vi "Lin_Rohner_Project.vi"() -> ()   [LabVIEW 2019]
uses:
  <vilib>/Platform/TimedLoop/XDataNode/timing_clust.ctl
  <vilib>/Platform/TimedLoop/XDataNode/nitl_modes.ctl
  <vilib>/Platform/TimedLoop/XDataNode/wakeup.ctl
  <vilib>/Analysis/3filter.llb/Filter Passband Type.ctl
  <vilib>/DAQmx/write.llb/DAQmx Write (Analog DBL 1Chan 1Samp).vi
  <vilib>/DAQmx/read.llb/DAQmx Read (Analog 1D DBL NChan 1Samp).vi
  <vilib>/DAQmx/create/channels.llb/DAQmx Create Channel (AO-Voltage-Basic).vi
  <vilib>/DAQmx/miscellaneous.llb/DAQmx Fill In Error Info.vi
  <vilib>/DAQmx/create/channels.llb/DAQmx Create Channel (AI-Voltage-Basic).vi
  <vilib>/platform/TimedLoop/XDataNode/XDataNode.xnode
  <vilib>/Platform/TimedLoop/XDataNode/XDNodeRunTimeDep.lvlib
  <vilib>/ptbypt/NI_PtbyPt.lvlib
  <vilib>/Analysis/NI_AALBase.lvlib
panel:
  in  "Force Feedback":bool
  in  "Choose a Controller(Turn them ON first!!!)":bool
  out "Force Feedback Control Voltage":dbl
  out "Force Feedback Control Voltage":dbl(graph)
  in  "low cutoff freq: force sensor":dbl=0.125 format="%0.3f"
  out "Filtered Paddle Angular acce(tachometer) [rad/s^2]":dbl(graph)
  out "Filtered Paddle Angular acce(tachometer) [rad/s^2]":dbl
  in  "low cutoff freq: paddle angular acce":dbl=0.125 format="%0.3f"
  out "Filtered Torque [Nm]":dbl
  out "Filtered Torque [Nm]":dbl(graph)
  out "Filtered Paddle Angular Velocity(tachometer) [rad/s]":dbl
  out "Filtered Paddle Angular Velocity(tachometer) [rad/s] 2":dbl(graph)
  in  "low cutoff freq: paddle angular velocity(tachometer)":dbl=0.125 format="%0.3f"
  out "Angular Position [deg]":dbl
  out "Angular Position [deg]":dbl(knob) scale=-32.5..32.5
  in  "B":dbl
  in  "K":dbl
  in  "Virtual Wall":bool
  in  "Position Filter":bool
  out "Compensation Voltage":dbl
  out "Compensation Voltage":dbl(graph)
  out "Gravity Compesation":dbl
  out "Friction Compensation":dbl
  in  "Friction Compensation":bool
  in  "Gravaty Compensation":bool
  out "Friction Compensation":dbl(graph)
  out "Gravity Compesation":dbl(graph)
  in  "low cutoff freq: Position":dbl=0.125 format="%0.3f"
  in  "stop":bool
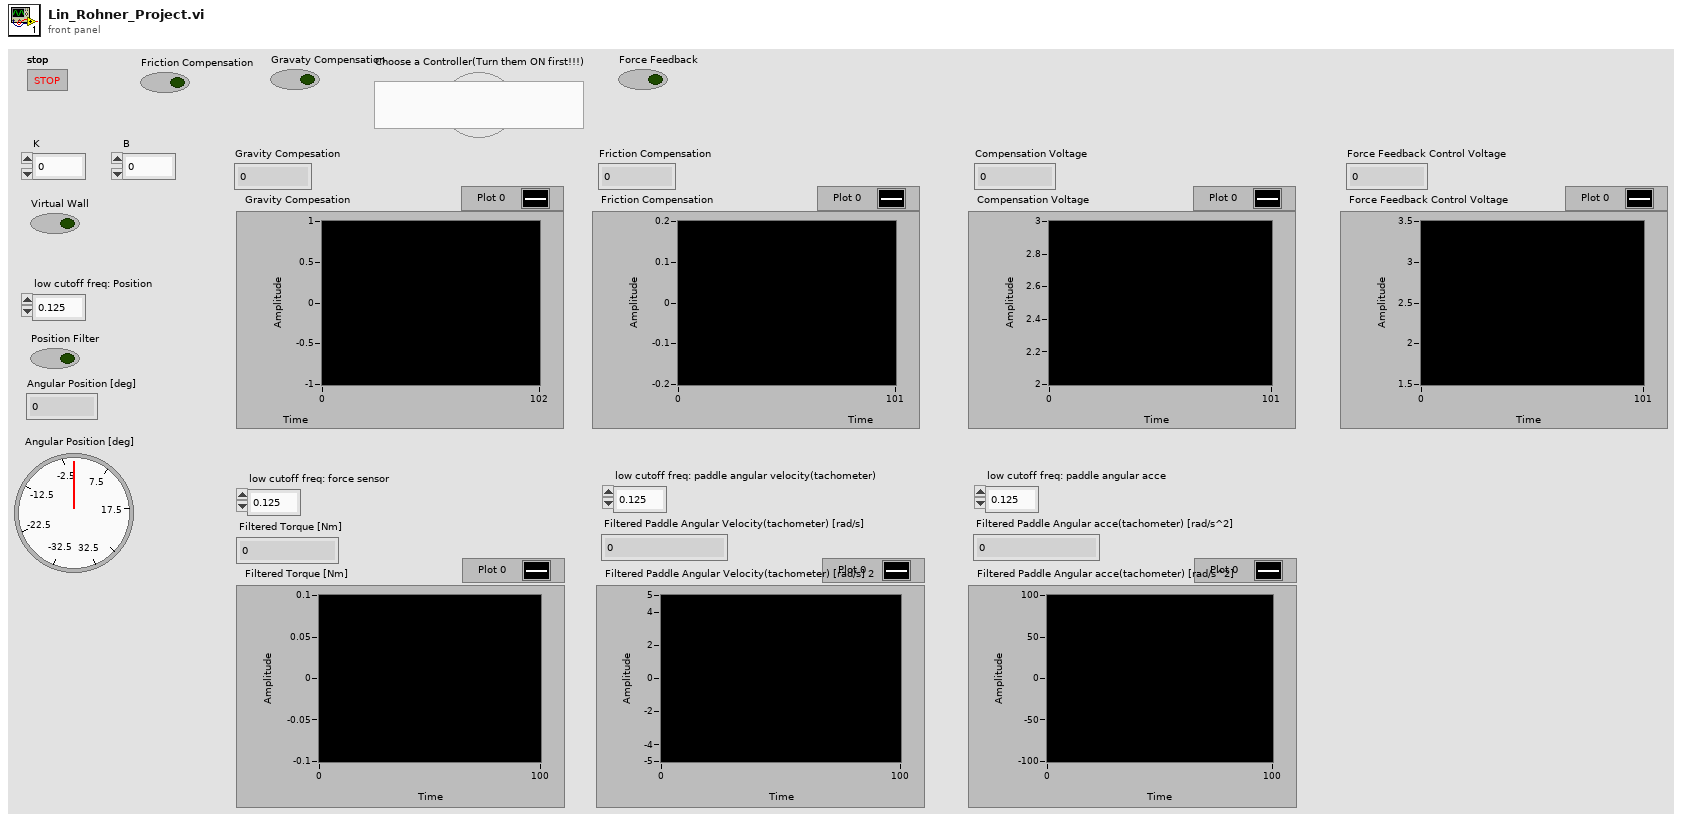
[diagram p1: front panel]
types:
  T1 = typedef "NI_AALBase.lvlib/Filter Passband Type.ctl" = enum32{"Lowpass", "Highpass", "Bandpass", "Bandstop"}
  T2 = typedef "XDNodeRunTimeDep.lvlib/timing_clust.ctl" = cluster{"Expected End [f-1]":u64, "Actual End [f-1]":u64, "Finished Late? [f-1]":bool, "Expected End [i-1]":u64, "Actual End [i-1]":u64, "Finished Late? [i-1]":bool, "Expected Start [i]":u64, "Actual Start [i]":u64, "Expected Start [f]":u64, "Actual Start [f]":u64, "Source Name":string, "Structure Name":string, "Period":i64, "Deadline":i64, "Offset":i64, "Start":i64, "Priority":i32, "Timeout":i32, "Mode":T3, "Wakeup Reason":T4, "Error":errorcluster, "Source Type":string, "Secondary Source Type":string, "Global End Time":u64, "Global Start Time":u64, "Frame Duration":u64, "Iteration Duration":u64, "Assigned CPU":i32, "I/O Scan Engine Mode":u32}
  T3 = typedef "XDNodeRunTimeDep.lvlib/nitl_modes.ctl" = enum32{"No Change", "Process missed periods, maintain original phase", "Discard missed periods, maintain original phase", "Process missed periods, ignore original phase", "Discard missed periods, ignore original phase"}
  T4 = typedef "XDNodeRunTimeDep.lvlib/wakeup.ctl" = enum32{"Normal", "Aborted", "Asynchronous wakeup", "Timing source error", "Timed loop error", "Timeout"}
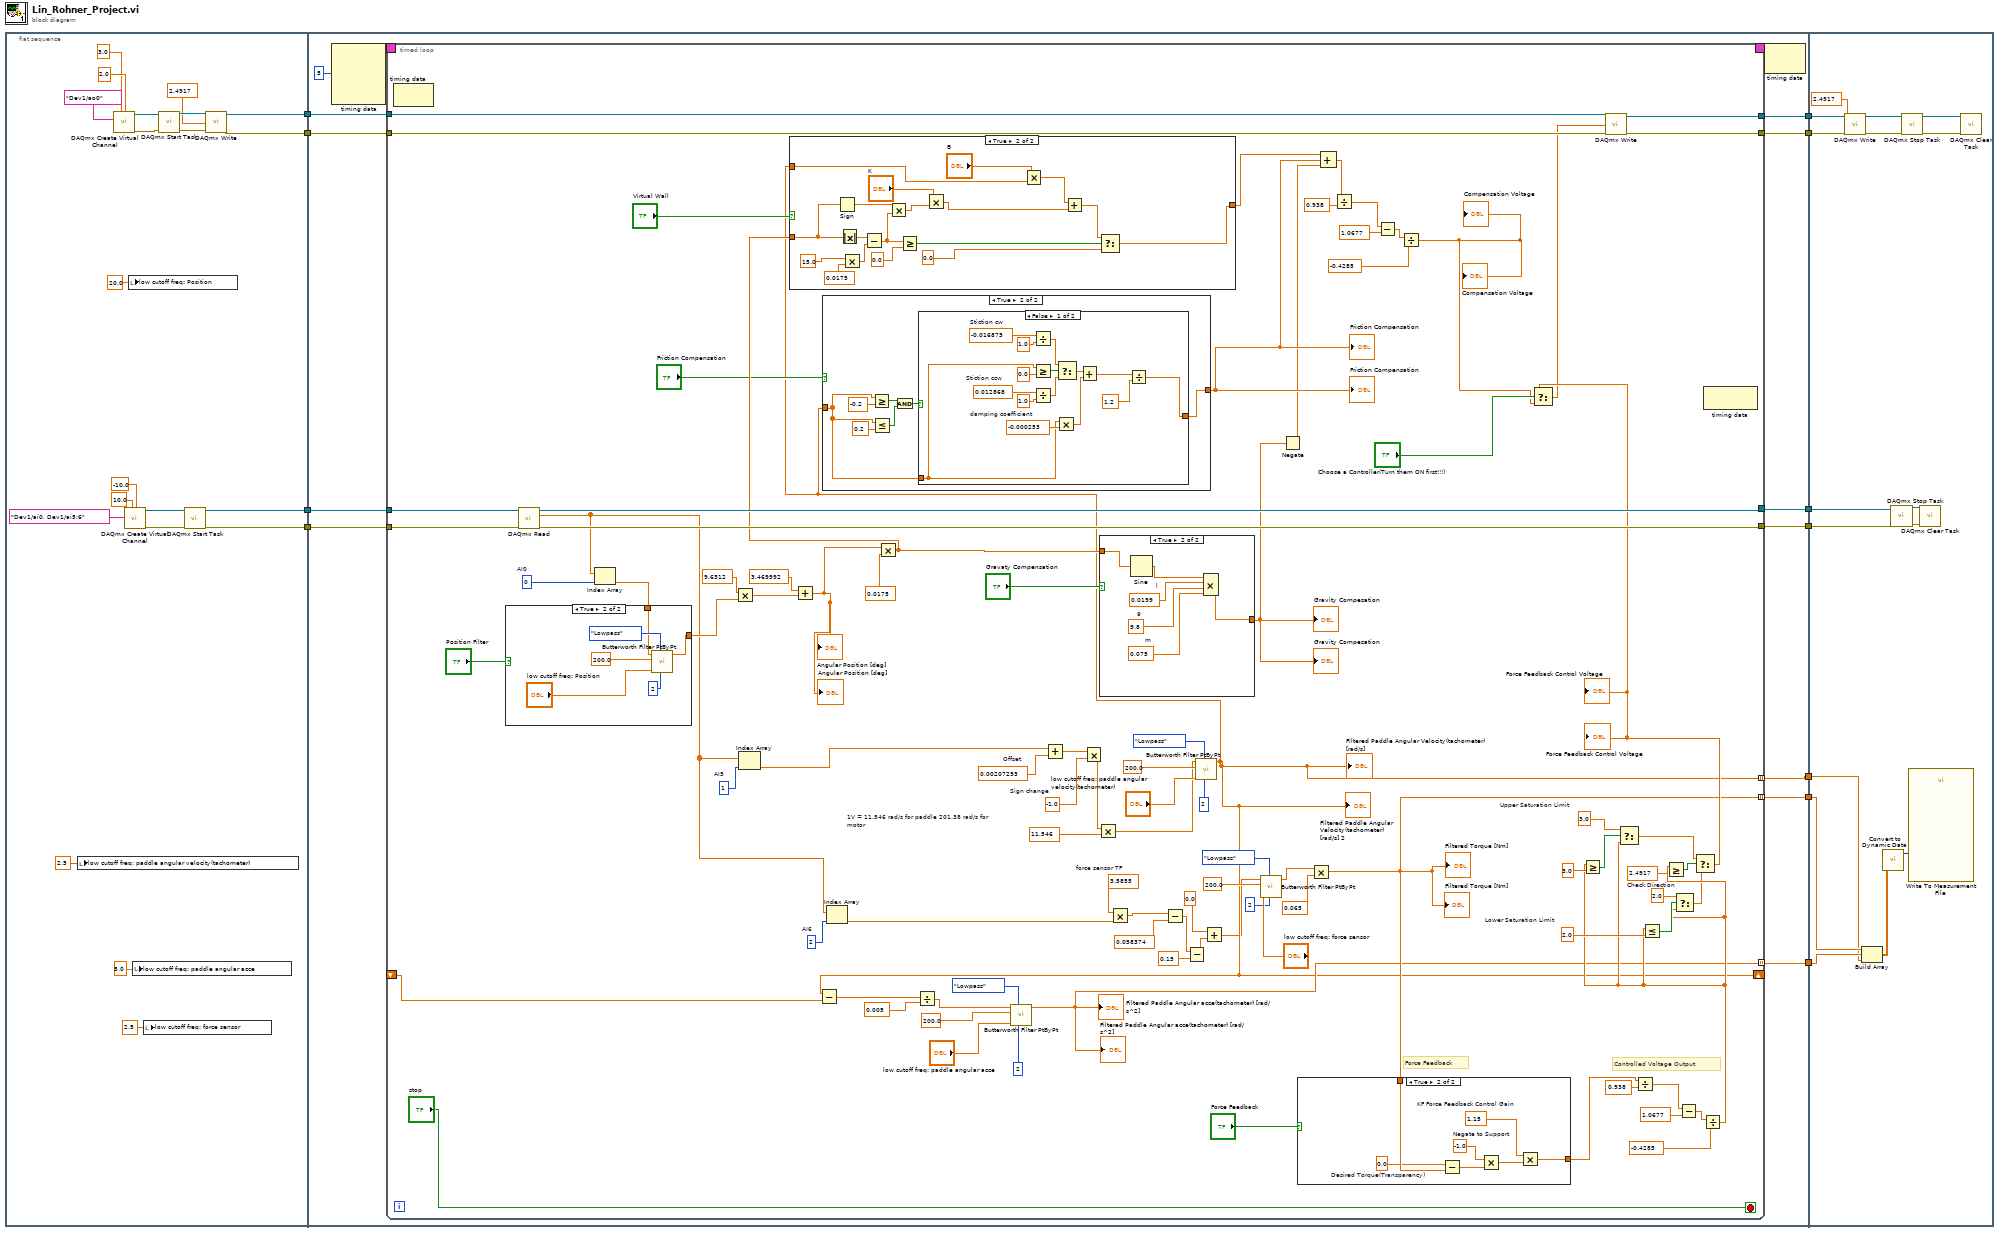
[diagram p0: block diagram]
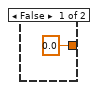
[diagram p2: hidden frame]
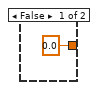
[diagram p3: hidden frame]
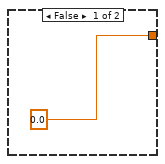
[diagram p5: hidden frame]
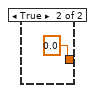
[diagram p6: hidden frame]
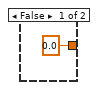
[diagram p7: hidden frame]
diagram:
  n1 = flat-sequence {
    tunnel: [w30] -> w11
    tunnel: [w29] -> w10
    tunnel: [w18] -> w9
    tunnel: [w17] -> w8
    tunnel: w11 -> [w43]
    tunnel: w10 -> [w42]
    tunnel: w9 -> [w41]
    tunnel: w8 -> [w40]
    tunnel: [w39] -> w7
    tunnel: [w38] -> w6
    tunnel: [w37] -> w5
    tunnel: [w36] -> w4
    tunnel: [w35] -> w3
    tunnel: [w34] -> w2
    tunnel: [w33] -> w1
    tunnel: w7 -> [w220]
    tunnel: w6 -> [w219]
    tunnel: w5 -> [w218]
    tunnel: w4 -> [w217]
    tunnel: w3 -> [w216]
    tunnel: w2 -> [w215]
    tunnel: w1 -> [w214]
    frame #0 {
      n2 = local write "low cutoff freq: paddle angular velocity(tachometer)"(2.5 ("low cutoff freq: paddle angular velocity(tachometer)")) -> ()
      n3 = call-poly <vilib>:"DAQmx Create Virtual Channel.vi"("maximum value"=3.0, "minimum value"=2.0, "physical channels"=tag "Dev1/ao0") -> ("task out"=w32:refnum<k21>, "error out"=w28:errorcluster)  [unwired: 11 in]
      n4 = call-poly <vilib>:"DAQmx Create Virtual Channel.vi"("maximum value"=10.0, "minimum value"=-10.0, "physical channels"=tag "Dev1/ai0, Dev1/ai5:6") -> ("task out"=w19:refnum<k21>, "error out"=w20:errorcluster)  [unwired: 11 in]
      n5 = local write "low cutoff freq: Position"(20.0 ("low cutoff freq: Position")) -> ()
      n6 = local write "low cutoff freq: paddle angular acce"(5.0 ("low cutoff freq: paddle angular acce")) -> ()
      n7 = local write "low cutoff freq: force sensor"(2.5 ("low cutoff freq: force sensor")) -> ()
      n8 = call <vilib>:"DAQmx Start Task.vi"("task/channels in"=w32, "error in"=w28) -> ("task out"=w31:refnum<k21>, "error out"=w27:errorcluster)  [unwired: 12 in]
      n9 = call <vilib>:"DAQmx Start Task.vi"("task/channels in"=w19, "error in"=w20) -> ("task out"=w18:refnum<k21>, "error out"=w17:errorcluster)  [unwired: 12 in]
      n10 = call-poly <vilib>:"DAQmx Write.vi"("task/channels in"=w31, "data"=2.4917, "error in"=w27) -> ("task out"=w30:refnum<k21>, "error out"=w29:errorcluster)  [unwired: 10 in, 1 out]
    }
    frame #1 {
      n11 = node-c288(i64 5 ("Period")) -> (w46:T2)  [unwired: 3 in]
      n12 = timed-loop {
        timing: w46 -> [_]
        timing-out: [_] -> w45
        tunnel: w43 -> [w136]
        tunnel: w42 -> [w135]
        tunnel: w41 -> [w134]
        tunnel: w40 -> [w133]
        tunnel: [w130] -> w39
        tunnel: [w129] -> w38
        tunnel: [w132] -> w37
        tunnel: [w131] -> w36
        shift-right: [w50] -> _
        shift-left: _ -> [w88]
        tunnel: [w52] -> w35 mode=indexing
        tunnel: [w51] -> w34 mode=indexing
        tunnel: [w50] -> w33 mode=indexing
        stop <- "stop" stop-if-true
        w61 = 2.4917  # Check Direction
        w65 = 2.0  # Lower Saturation Limit
        w68 = 3.0  # Upper Saturation Limit
        w94 = 3.5855  # force sensor TF
        w96 = 2  # AI6
        w103 = 11.546  # 1V = 11.546 rad/s for paddle 201.38 rad/s for motor
        w105 = -1.0  # Sign change
        w107 = 0.00207293  # Offset
        w109 = 1  # AI5
        w111 = 0  # AI0
        # "Controlled Voltage Output"
        # "Force Feedback"
        n13 = node-c288() -> ()  [unwired: 1 in, 1 out]
        n14 = call-poly <vilib>:"DAQmx Read.vi"("task/channels in"=w134, "error in"=w133) -> ("task out"=w132:refnum<k21>, "data"=w91:dbl[], "error out"=w131:errorcluster)  [unwired: 11 in]
        n15 = Index Array(array=w91, index=w111) -> (element=w110:dbl)
        n16 = case shown="True" "Position Filter" {
          tunnel: [w168 w171] -> w137
          tunnel: w110 -> [w168 w169]
          frame False {
          }
          frame True {
            n17 = call <vilib>:"Butterworth Filter PtByPt.vi"("order"=2, "filter type"=Filter_Passband_Type."Lowpass", "low cutoff freq: fl"="low cutoff freq: Position", "sampling freq: fs"=200.0, "x"=w169) -> ("Filtered x"=w171:dbl)  [unwired: 4 in, 1 out]
          }
        }
        n18 = Multiply(x=9.6312, y=w137) -> (x*y=w139:dbl)
        n19 = Index Array(array=w91, index=w109) -> (element=w108:dbl)
        n20 = Add(x=3.469992, y=w139) -> (x+y=w112:dbl)
        "Angular Position [deg]" <- w112
        "Angular Position [deg]" <- w112
        n21 = Index Array(array=w91, index=w96) -> (element=w95:dbl)
        n22 = Multiply(x=w112, y=0.0175) -> (x*y=w113:dbl)
        n23 = Add(x=w108, y=w107) -> (x+y=w106:dbl)
        n24 = Multiply(x=w106, y=w105) -> (x*y=w104:dbl)
        n25 = Multiply(x=w104, y=w103) -> (x*y=w98:dbl)
        n26 = case shown="True" "Gravaty Compensation" {
          tunnel: [0.0 w201] -> w120
          tunnel: w113 -> [_ w200]
          frame False {
          }
          frame True {
            w202 = 0.075  # m
            w203 = 9.8  # g
            w204 = 0.0199  # l
            n27 = Sine(x=w200) -> (sin(x)=w205:dbl)
            n28 = Compound Arithmetic op=MULTIPLY(w205, w204, w203, w202) -> (w201:dbl)
          }
        }
        "Gravity Compesation" <- w120
        "Gravity Compesation" <- w120
        n29 = Multiply(x=w94, y=w95) -> (x*y=w93:dbl)
        n30 = Subtract(x=w93, y=0.058374) -> (x-y=w89:dbl)
        n31 = Subtract(x=w89, y=0.15) -> (x-y=w49:dbl)
        n32 = call <vilib>:"Butterworth Filter PtByPt.vi"("order"=2, "filter type"=Filter_Passband_Type."Lowpass", "low cutoff freq: fl"="low cutoff freq: paddle angular velocity(tachometer)", "sampling freq: fs"=200.0, "x"=w98) -> ("Filtered x"=w50:dbl)  [unwired: 4 in, 1 out]
        "Filtered Paddle Angular Velocity(tachometer) [rad/s] 2" <- w50
        "Filtered Paddle Angular Velocity(tachometer) [rad/s]" <- w50
        n33 = case shown="True" "Virtual Wall" {
          tunnel: w113 -> [_ w163]
          tunnel: w50 -> [_ w159]
          tunnel: [0.0 w155] -> w115
          frame False {
          }
          frame True {
            n34 = Sign(1:w163) -> (0:w162:dbl)
            n35 = Absolute Value(x=w163) -> (abs(x)=w166:dbl)
            n36 = Multiply(x=15.0 ("y"), y=0.0175) -> (x*y=w150:dbl)
            n37 = Subtract(x=w166, y=w150) -> (x-y=w161:dbl)
            n38 = Multiply(x=w162, y=w161) -> (x*y=w160:dbl)
            n39 = Greater Or Equal?(x=w161, y=0.0) -> (x >= y?=w164:bool)
            n40 = Multiply(x="K", y=w160) -> (x*y=w157:dbl)
            n41 = Multiply(x="B", y=w159) -> (x*y=w158:dbl)
            n42 = Add(x=w158, y=w157) -> (x+y=w156:dbl)
            n43 = Select(t=w156, s=w164, f=0.0) -> (s? t:f=w155:dbl)
          }
        }
        n44 = Subtract(x=w50, y=w88) -> (x-y=w87:dbl)
        n45 = case shown="True" "Friction Compensation" {
          tunnel: [0.0 ("f") w177] -> w117
          tunnel: w50 -> [_ w176]
          frame False {
          }
          frame True {
            n46 = Greater Or Equal?(x=w176, y=-0.2) -> (x >= y?=w180:bool)
            n47 = Less Or Equal?(x=w176, y=0.2) -> (x <= y?=w179:bool)
            n48 = And(x=w180, y=w179) -> (x .and. y?=w178:bool)
            n49 = case shown="False" w178 {
              tunnel: [w184 0.0 ("y")] -> w177
              tunnel: w176 -> [w193 _]
              frame False {
                w195 = -0.000253  # damping coefficient
                w191 = 0.012868  # Stiction ccw
                w188 = -0.016875  # Stiction cw
                n50 = Divide(x=w188, y=1.0) -> (x/y=w187:dbl)
                n51 = Greater Or Equal?(x=w193, y=0.0) -> (x >= y?=w196:bool)
                n52 = Divide(x=w191, y=1.0) -> (x/y=w190:dbl)
                n53 = Multiply(x=w193, y=w195) -> (x*y=w194:dbl)
                n54 = Select(t=w187, s=w196, f=w190) -> (s? t:f=w192:dbl)
                n55 = Add(x=w192, y=w194) -> (x+y=w185:dbl)
                n56 = Divide(x=w185, y=1.2) -> (x/y=w184:dbl)
              }
              frame True {
              }
            }
          }
        }
        "Friction Compensation" <- w117
        "Friction Compensation" <- w117
        n57 = Divide(x=w87, y=0.005) -> (x/y=w85:dbl)
        n58 = call <vilib>:"Butterworth Filter PtByPt.vi"("order"=2, "filter type"=Filter_Passband_Type."Lowpass", "low cutoff freq: fl"="low cutoff freq: paddle angular acce", "sampling freq: fs"=200.0, "x"=w85) -> ("Filtered x"=w51:dbl)  [unwired: 4 in, 1 out]
        "Filtered Paddle Angular acce(tachometer) [rad/s^2]" <- w51
        "Filtered Paddle Angular acce(tachometer) [rad/s^2]" <- w51
        n59 = Add(x=0.0, y=w49) -> (x+y=w47:dbl)
        n60 = call <vilib>:"Butterworth Filter PtByPt.vi"("order"=2, "filter type"=Filter_Passband_Type."Lowpass", "low cutoff freq: fl"="low cutoff freq: force sensor", "sampling freq: fs"=200.0, "x"=w47) -> ("Filtered x"=w76:dbl)  [unwired: 4 in, 1 out]
        n61 = Negate(x=w120) -> (-x=w116:dbl)
        n62 = Multiply(x=w76, y=0.065) -> (x*y=w52:dbl)
        "Filtered Torque [Nm]" <- w52
        "Filtered Torque [Nm]" <- w52
        n63 = case shown="True" "Force Feedback" {
          tunnel: w52 -> [_ w148]
          tunnel: [0.0 w142] -> w69
          frame False {
          }
          frame True {
            w143 = 1.15  # KF Force Feedback Control Gain
            w145 = -1.0  # Negate to Support
            w147 = 0.0  # Desired Torque(Transparency)
            n64 = Subtract(x=w147, y=w148) -> (x-y=w146:dbl)
            n65 = Multiply(x=w145, y=w146) -> (x*y=w144:dbl)
            n66 = Multiply(x=w143, y=w144) -> (x*y=w142:dbl)
          }
        }
        n67 = Compound Arithmetic op=ADD(w115, w117, w116) -> (w114:dbl)
        n68 = Divide(x=w114, y=0.938) -> (x/y=w124:dbl)
        n69 = Subtract(x=w124, y=1.0677) -> (x-y=w122:dbl)
        n70 = Divide(x=w122, y=-0.4285) -> (x/y=w56:dbl)
        "Compensation Voltage" <- w56
        "Compensation Voltage" <- w56
        n71 = Divide(x=w69, y=0.938) -> (x/y=w73:dbl)
        n72 = Subtract(x=w73, y=1.0677) -> (x-y=w71:dbl)
        n73 = Divide(x=w71, y=-0.4285) -> (x/y=w62:dbl)
        n74 = Greater Or Equal?(x=w62, y=3.0) -> (x >= y?=w66:bool)
        n75 = Select(t=w68, s=w66, f=w62) -> (s? t:f=w59:dbl)
        n76 = Less Or Equal?(x=w62, y=w65) -> (x <= y?=w64:bool)
        n77 = Greater Or Equal?(x=w62, y=w61) -> (x >= y?=w60:bool)
        n78 = Select(t=2.0, s=w64, f=w62) -> (s? t:f=w58:dbl)
        n79 = Select(t=w59, s=w60, f=w58) -> (s? t:f=w55:dbl)
        "Force Feedback Control Voltage" <- w55
        "Force Feedback Control Voltage" <- w55
        n80 = Select(t=w55, s="Choose a Controller(Turn them ON first!!!)", f=w56) -> (s? t:f=w54:dbl)
        n81 = call-poly <vilib>:"DAQmx Write.vi"("task/channels in"=w136, "data"=w54, "error in"=w135) -> ("task out"=w130:refnum<k21>, "error out"=w129:errorcluster)  [unwired: 10 in, 1 out]
        n82 = node-c288() -> ()  [unwired: 1 in, 1 out]
      }
      n83 = node-c288(w45) -> ()  [unwired: 1 out]
    }
    frame #2 {
      n84 = call-poly <vilib>:"DAQmx Write.vi"("task/channels in"=w220, "data"=2.4917, "error in"=w219) -> ("task out"=w227:refnum<k21>, "error out"=w224:errorcluster)  [unwired: 10 in, 1 out]
      n85 = Build Array(w216, w215, w214) -> (w213:dbl[][])
      n86 = call "Convert to Dynamic Data"("2D Array"=w213) -> ("Dynamic Data Type"=w212:dynamicdata)  [unwired: 3 in]
      n87 = call <vilib>:"DAQmx Stop Task.vi"("task/channels in"=w218, "error in"=w217) -> ("task out"=w221:refnum<k21>, "error out"=w222:errorcluster)  [unwired: 12 in]
      n88 = call <vilib>:"DAQmx Stop Task.vi"("task/channels in"=w227, "error in"=w224) -> ("task out"=w226:refnum<k21>, "error out"=w225:errorcluster)  [unwired: 12 in]
      n89 = call "Write To Measurement File"("Signals"=w212) -> ()  [unwired: 16 in, 3 out]
      n90 = call <vilib>:"DAQmx Clear Task.vi"("task in"=w221, "error in"=w222) -> ()  [unwired: 13 in, 1 out]
      n91 = call <vilib>:"DAQmx Clear Task.vi"("task in"=w226, "error in"=w225) -> ()  [unwired: 13 in, 1 out]
    }
  }
